vi "查找匹配关闭标识符.vi"(8 "error in":errorcluster caption="错误输入", 10 "element name":string caption="元素名", 11 "XML string in":string caption="XML字符串输入") -> (0 "error out":errorcluster caption="错误输出", 1 "text after end tag":string caption="结束标识符之后文本", 2 "close tag":string caption="关闭标识符", 3 "string before end tag":string caption="结束标识符之前字符串", 4 "offset past close tag":i32 caption="关闭标识符偏移量")   [LabVIEW 2017]
panel:
  in  "error message":string="结束标识符未找到\n" caption="错误信息"
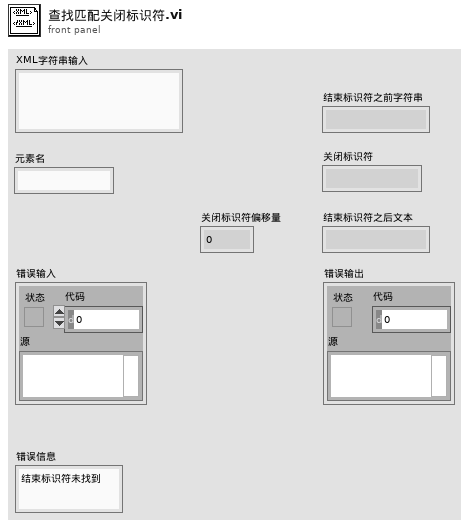
[diagram p1: front panel]
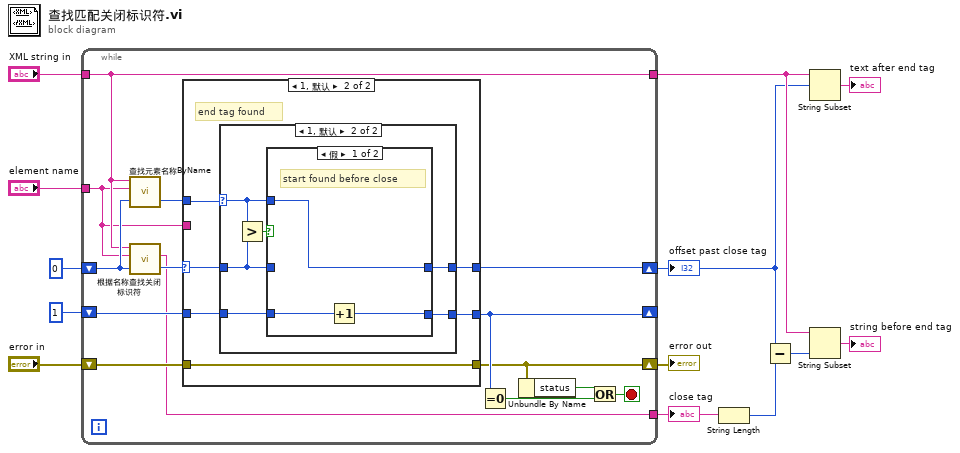
[diagram p0: block diagram]
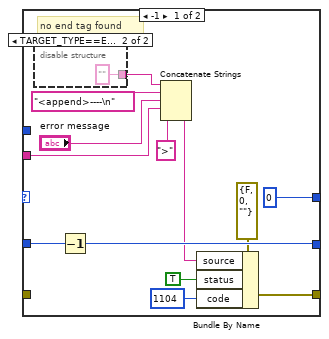
[diagram p2: hidden frame]
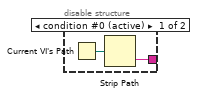
[diagram p3: hidden frame]
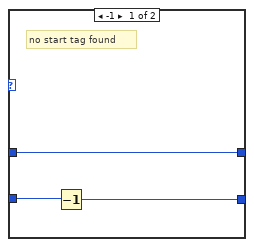
[diagram p4: hidden frame]
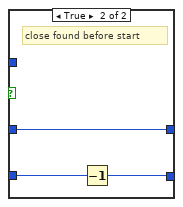
[diagram p5: hidden frame]
diagram:
  n1 = while {
    tunnel: "XML string in" -> [w19]
    tunnel: "element name" -> [w17]
    shift-right: [w15] -> w13
    shift-left: "error in" -> [w27]
    shift-right: [w22] -> w2
    shift-left: 0 ("offset past match") -> [w24]
    shift-right: [w20] -> _
    shift-left: 1 ("offset past match") -> [w26]
    tunnel: [w18] -> w7
    tunnel: [w19] -> w5
    stop <- w16 stop-if-true
    n2 = call "查找元素名称ByName.vi"("offset (0)"=w24, "Element Name"=w17, "string"=w19) -> ("offset past match"=w23:i32)  [unwired: 5 in, 3 out]
    n3 = call "根据名称查找关闭标识符.vi"("offset (0)"=w24, "close Tag"=w17, "string"=w19) -> ("match close tag"=w18:string, "offset past close tag"=w25:i32)  [unwired: 5 in, 2 out]
    n4 = case shown="1, 默认" w25 {
      selector: w25 -> [_ w48]
      tunnel: w23 -> [_ w45]
      tunnel: [0 ("offset past match") w49] -> w22
      tunnel: w26 -> [w40 w47]
      tunnel: [w39 w46] -> w20
      tunnel: w27 -> [_ w44]
      tunnel: [w35 w44] -> w15
      tunnel: w17 -> [w29 _]
      frame -1 {
        # "no end tag found"
        n5 = disable-structure shown="TARGET_TYPE==Embedded||TARGET_TYPE==PocketPC" {
          disable-tunnel: [w41 "" ("name")] -> w33
          frame condition #0 (active) {
            n6 = Current VI's Path() -> (path=w42:path)
            n7 = Strip Path(path=w42) -> (name=w41:string)  [unwired: 1 out]
          }
          frame condition #1 {
          }
        }
        n8 = Decrement(x=w40) -> (x-1=w39:i32)
        n9 = Concatenate Strings(w33, "<append>----\n" ("string"), "error message", w29, ">" ("string")) -> (w31:string)
        n10 = Bundle By Name(cluster=errorcluster {"status"=FALSE, "code"=0, "source"=""} ("error in"), "source"=w31, "status"=TRUE, "code"=1104) -> (w35:errorcluster)
      }
      frame 1, Default {
        # "end tag found"
        n11 = case shown="1, 默认" w45 {
          selector: w45 -> [_ w53]
          tunnel: [w50 w57] -> w49
          tunnel: w48 -> [w50 w56]
          tunnel: w47 -> [w52 w55]
          tunnel: [w51 w54] -> w46
          frame -1 {
            # "no start tag found"
            n12 = Decrement(x=w52) -> (x-1=w51:i32)
          }
          frame 1, Default {
            n13 = Greater?(x=w53, y=w56) -> (0:w58:bool)
            n14 = case shown="假" w58 {
              tunnel: w56 -> [_ w62]
              tunnel: w53 -> [w59 _]
              tunnel: [w59 w62] -> w57
              tunnel: w55 -> [w61 w64]
              tunnel: [w60 w63] -> w54
              frame False {
                # "start found before close"
                n15 = Increment(x=w61) -> (x+1=w60:i32)
              }
              frame True {
                # "close found before start"
                n16 = Decrement(x=w64) -> (x-1=w63:i32)
              }
            }
          }
        }
      }
    }
    n17 = Equal To 0?(x=w20) -> (x = 0?=w21:bool)
    n18 = Unbundle By Name(w15) -> ("status"=w14:bool)
    n19 = Or(x=w14, y=w21) -> (x .or. y?=w16:bool)
  }
  "error out" <- w13
  "offset past close tag" <- w2
  "close tag" <- w7
  n20 = String Length(string=w7) -> (length=w3:i32)
  n21 = Subtract(x=w2, y=w3) -> (x-y=w6:i32)
  n22 = String Subset(string=w5, offset (0)=w2) -> (substring=→"text after end tag":string)  [unwired: 1 in]
  n23 = String Subset(string=w5, length (rest)=w6) -> (substring=→"string before end tag":string)  [unwired: 1 in]
